vi "Plot Helper (Matrix).vi"(0 "3D Plot lvclass Array in":refnum<class "3D Plot Datatype.lvclass">[](array[class]), 1 "Nx matrix":sgl[][](array[numeric]), 2 "Ny matrix":sgl[][](array[numeric]), 3 "Nz matrix":sgl[][](array[numeric]), 5 "x matrix":sgl[][](array[numeric]), 7 "y matrix":sgl[][](array[numeric]), 9 "z matrix":sgl[][](array[numeric]), 11 "error in (no error)":errorcluster, 14 "Plot ID":i32) -> (4 "3D Plot lvclass Array out":refnum<class "3D Plot Datatype.lvclass">[](array[class]), 15 "error out":errorcluster)   [LabVIEW 2020, in "3D Quiver Datatype.lvclass"]
doc: "Graphs a plot of normal vectors. Multiple references to this VI generate multiple plots for the same graph."
uses:
  <vilib>/Math Plots/3D Math Plots/3D Quiver/3D Quiver Datatype/3D Quiver Datatype.lvclass
  <vilib>/Math Plots/3D Math Plots/3D Plot/3D Plot Datatype/3D Plot Datatype.lvclass
  e:/builds/penguin/labview/branches/2020/dev/dist/vi.lib/Math Plots/3D Math Plots/3D Plot/3D Plot Datatype/3D Plot Datatype.lvclass
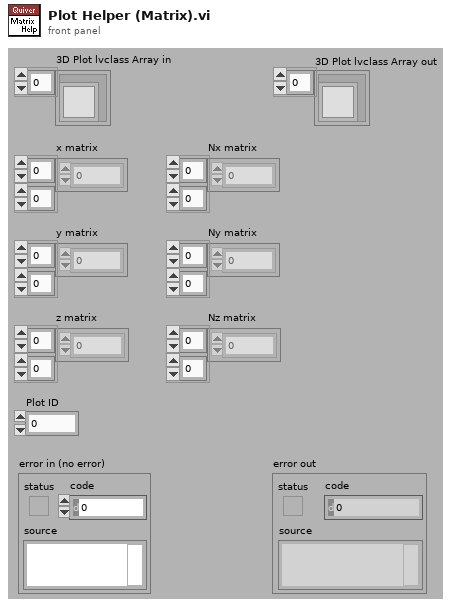
[diagram p1: front panel]
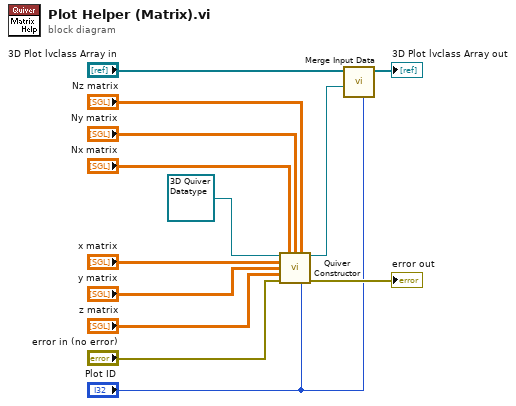
[diagram p0: block diagram]
diagram:
  n1 = call <vilib>:"Quiver Constructor.vi"("3D Quiver Datatype.lvclass in"=refnum<class "3D Quiver Datatype.lvclass"> refnum ("3D Quiver Datatype.lvclass"), "Nx Matrix"="Nx matrix", "Ny Matrix"="Ny matrix", "Nz matrix"="Nz matrix", "x vector"="x matrix", "y vector"="y matrix", "z matrix"="z matrix", "error in (no error)"="error in (no error)", "Plot ID"="Plot ID") -> ("3D Quiver Datatype.lvclass out"=w5:refnum<class "3D Quiver Datatype.lvclass">, "error out"=→"error out":errorcluster)  [unwired: 5 out]
  n2 = call <vilib>:"Merge Input Data.vi"("Plot ID"="Plot ID", "3D Plot lvclass in"=w5, "3D Plot lvclass Array in"="3D Plot lvclass Array in") -> ("3D Plot lvclass Array out"=→"3D Plot lvclass Array out":refnum<class "3D Plot Datatype.lvclass">[])  [unwired: 8 out]
